vi "Read Cluster Array.vi"(8 "error in (no error)":errorcluster, 9 "Regular Expression":string, 10 "Arr Refnum":refnum<vi>, 11 "file refnum":T6=refnum) -> (0 "error out":errorcluster)   [LabVIEW 2021, in "CANOpen Addon System Explorer.lvlib"]
uses:
  CANOpen Addon System Explorer.lvlib
  <vilib>/Utility/config.llb/Config Data RefNum.ctl
  control/OD Entry.ctl
  control/Object Type.ctl
  control/Data Type.ctl
  control/Access Type.ctl
  control/OD Cateory.ctl
  <vilib>/Utility/config.llb/NI_LVConfig.lvlib
panel:
  out "OD Entry":T1={"index"=0, "sub-index"=0, "Level"=10, "ObjectType"=0, "DataType"=0, "ParameterName"="", "LowLimit"="", "HighLimit"="", "AccessType"=0, "DefaultValue"="", "PDOMapping"=FALSE, "SubNumber"=0, "ObjFlags"=0, "Category"=enum."Mandatory"} {"AccessType" items=["", "ro", "wo", "rw", "const", "rwr", "rww"]; "DataType" items=[""=0, "BOOLEAN"=1, "INTEGER8"=2, "INTEGER16"=3, "INTEGER32"=4, "UNSIGNED8"=5, "UNSIGNED16"=6, "UNSIGNED32"=7, "REAL32"=8, "VISIBLE_STRING"=9, "OCTET_STRING"=10, "UNICODE_STRING"=11, "TIME_OF_DAY"=12, "TIME_DIFFERENCE"=13, "DOMAIN"=15, "INTEGER24"=16, "REAL64"=17, "INTEGER40"=18, "INTEGER48"=19, "INTEGER56"=20, "INTEGER64"=21, "UNSIGNED24"=22, "UNSIGNED40"=24, "UNSIGNED48"=25, "UNSIGNED56"=26, "UNSIGNED64"=27]; "ObjectType" items=[""=10, "NULL"=0, "DOMAIN"=2, "DEFTYPE"=5, "DEFSTRUCT"=6, "VAR"=7, "ARRAY"=8, "RECORD"=9]}
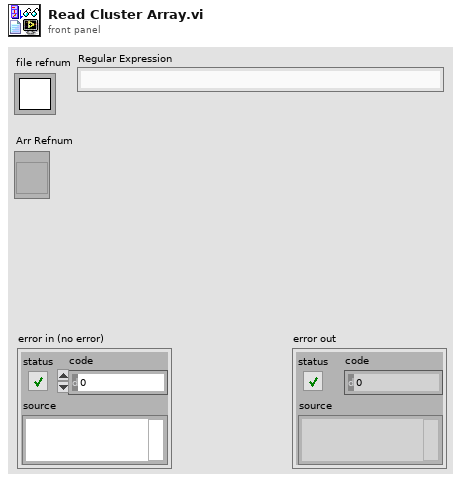
[diagram p1: front panel]
types:
  T1 = typedef "CANOpen Addon System Explorer.lvlib/OD Entry.ctl" = cluster{"index":u16, "sub-index":u8, "Level":u8, "ObjectType":T2, "DataType":T3, "ParameterName":string, "LowLimit":string, "HighLimit":string, "AccessType":T4, "DefaultValue":string, "PDOMapping":bool, "SubNumber":u8, "ObjFlags":u32, "Category":T5}
  T2 = typedef "CANOpen Addon System Explorer.lvlib/Object Type.ctl" = u16
  T3 = typedef "CANOpen Addon System Explorer.lvlib/Data Type.ctl" = u16
  T4 = typedef "CANOpen Addon System Explorer.lvlib/Access Type.ctl" = u16
  T5 = typedef "CANOpen Addon System Explorer.lvlib/OD Cateory.ctl" = enum16{"Mandatory", "Optional", "Manufacturer", ""}
  T6 = typedef "NI_LVConfig.lvlib/Config Data RefNum.ctl" = refnum<k1>
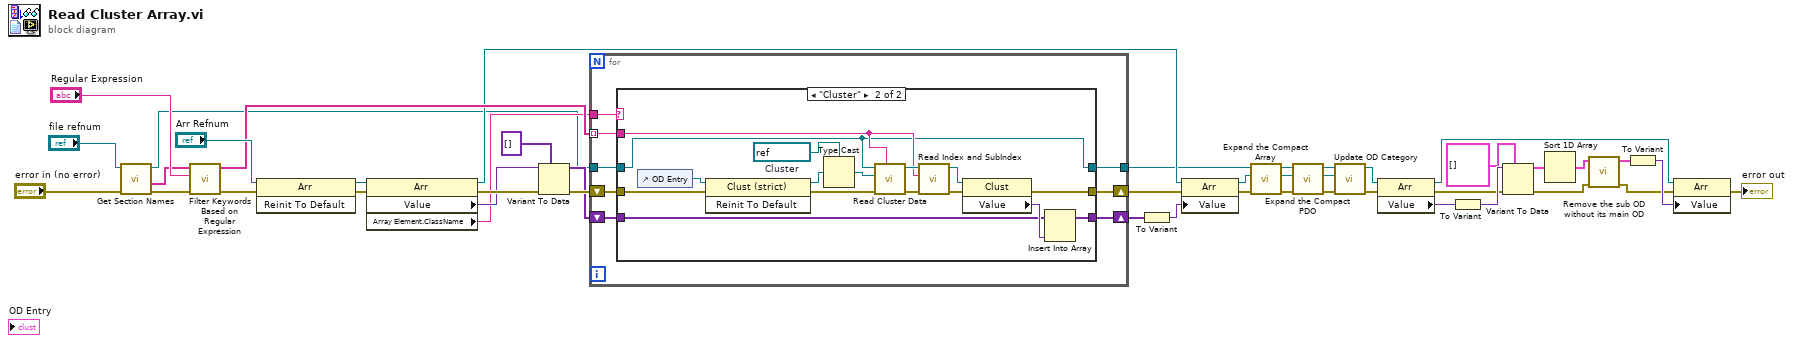
[diagram p0: block diagram]
diagram:
  n1 = call <vilib>:"Get Section Names.vi"("error in (no error)"="error in (no error)", "refnum"="file refnum") -> ("error out"=w29:errorcluster, "section names"=w27:string[], "refnum out"=w28:T6)  [unwired: 7 in]
  n2 = call "Filter Keywords Based on Regular Expression.vi"("error in (no error)"=w29, "Regular Expression"="Regular Expression", "Words"=w27) -> ("error out"=w43:errorcluster, "Filters Words"=w40:string[])  [unwired: 7 in]
  n3 = invoke class="Arr" method="Reinit To Default"(reference="Arr Refnum", error in=w43) -> (reference out=w41:refnum<vi>, error out=w42:errorcluster)  [unwired: 1 in, 1 out]
  n4 = property class="Arr"(reference=w41, error in=w42) -> (reference out=w34:refnum<vi>, error out=w39:errorcluster, "Value"=w36:variant, "Array Element.ClassName"=w33:string)
  n5 = Variant To Data(error in=w39, type=variant[] [], Variant=w36) -> (data=w35:variant[], error out=w38:errorcluster)
  n6 = for {
    shift-right: [w51] -> w10
    shift-left: w38 -> [w52]
    tunnel: w40 -> [w46] mode=indexing
    shift-right: [w49] -> w22
    shift-left: w35 -> [w50]
    tunnel: w28 -> [w48]
    tunnel: w33 -> [w47]
    tunnel: [w45] -> w19
    n7 = case shown="\"Cluster\"" w47 {
      tunnel: w52 -> [w55 w66]
      tunnel: [w55 w68] -> w51
      tunnel: w50 -> [w54 w69]
      tunnel: [w54 w67] -> w49
      tunnel: w48 -> [w53 w58]
      tunnel: w46 -> [_ w60]
      tunnel: [w53 w58] -> w45
      frame "others", Default {
      }
      frame "Cluster" {
        w71 = refnum<vi> refnum  # Cluster
        n8 = control-ref of="OD Entry"() -> (w59:refnum<vi>)
        n9 = invoke on="Invoke Node" class="Clust (strict)" method="Reinit To Default"(reference=w59, error in=w66) -> (reference out=w65:refnum<vi>, error out=w64:errorcluster)  [unwired: 1 in, 1 out]
        n10 = Type Cast(type=w71, x=w65) -> (*(type *) &x=w63:refnum<vi>)
        n11 = call "Read Cluster Data.vi"("Section Name"=w60, "error in (no error)"=w64, "Clust Refnum"=w63, "File Refnum"=w58) -> ("error out"=w62:errorcluster, "dup Clust Refnum"=w61:refnum<vi>)  [unwired: 6 in]
        n12 = call "Read Index and SubIndex.vi"("error in (no error)"=w62, "Section"=w60, "Clust Refnum"=w61) -> ("error out"=w57:errorcluster, "dup Clust Refnum"=w56:refnum<vi>)  [unwired: 7 in]
        n13 = property class="Clust"(reference=w56, error in=w57) -> (error out=w68:errorcluster, "Value"=w70:variant)  [unwired: 1 out]
        n14 = Insert Into Array(array=w69, new element=w70) -> (w67:variant[])  [unwired: 1 in]
      }
    }
  }
  n15 = To Variant(anything=w22) -> (Variant=w18:variant)
  n16 = property class="Arr"(reference=w34, error in=w10, "Value"=w18) -> (reference out=w20:refnum<vi>, error out=w21:errorcluster)
  n17 = call "Expand the Compact Array.vi"("error in (no error)"=w21, "Arr Refnum"=w20, "File Refnum"=w19) -> ("error out"=w13:errorcluster, "dup Arr Refnum"=w11:refnum<vi>, "dup File Refnum"=w12:T6)  [unwired: 6 in]
  n18 = call "Expand the Compact PDO.vi"("error in (no error)"=w13, "Arr Refnum"=w11, "File Refnum"=w12) -> ("error out"=w9:errorcluster, "dup File Refnum"=w5:T6, "dup Arr Refnum"=w7:refnum<vi>)  [unwired: 6 in]
  n19 = call "Update OD Category.vi"("error in (no error)"=w9, "file refnum"=w5, "Arr Refnum"=w7) -> ("error out"=w8:errorcluster, "dup Arr Refnum"=w6:refnum<vi>)  [unwired: 7 in]
  n20 = property class="Arr"(reference=w6, error in=w8) -> (reference out=w15:refnum<vi>, error out=w4:errorcluster, "Value"=w17:variant)
  n21 = To Variant(anything=w17) -> (Variant=w26:variant)
  n22 = Variant To Data(error in=w4, type=T1[] [], Variant=w26) -> (data=w24:T1[], error out=w2:errorcluster)
  n23 = Sort 1D Array(array=w24) -> (sorted array=w23:T1[])
  n24 = call "Remove the sub OD without its main OD.vi"("error in (no error)"=w2, "ODs in"=w23) -> ("error out"=w1:errorcluster, "ODs out"=w3:T1[])  [unwired: 8 in]
  n25 = To Variant(anything=w3) -> (Variant=w16:variant)
  n26 = property class="Arr"(reference=w15, error in=w1, "Value"=w16) -> (error out=→"error out":errorcluster)  [unwired: 1 out]
